vi "Ximea Camera Engine.vi"(0 "Ximea Notifier Name":string, 11 "Camera ID":string[](array[string])) -> ()   [LabVIEW 2016]
uses:
  Ximea Controls/Ximea ROI.ctl
  Ximea Controls/Ximea Parameters.ctl
  Ximea Controls/Ximea Parameter List.ctl
  xiLIB_64bit/xiLIB/xiCamLib/xiCam/PRM/PRM/PRM_v2.ctl
  Ximea Controls/Ximea Notifier Element.ctl
  Ximea Controls/Ximea Actions.ctl
  <vilib>/vision/Image Controls.llb/IMAQ Image.ctl
  Camera Controls/Camera IMAQ Key Info.ctl
panel:
  in  "Use Display Module":bool
  in  "Quit":bool
  in  "Record":bool
  in  "Preview":bool
  out "Acquisition Loop":i32
  in  "Get Param":bool
  in  "Set Param":bool
  in  "Ximea  Parameter":T1
  in  "Get ROI":bool
  in  "Set ROI":bool
  in  "ROI Setup":T3
  out "Acquisition Frame":u32
  out "Serial No.":string
  out "Device Name":string
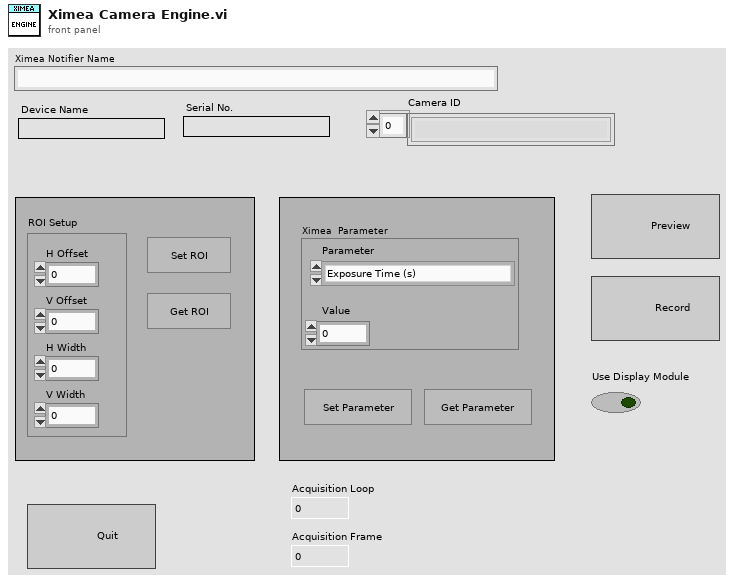
[diagram p1: front panel]
types:
  T1 = typedef "Ximea Parameters.ctl" = cluster{"Parameter":T2, "Value":sgl}
  T2 = typedef "Ximea Parameter List.ctl" = enum16{"Exposure Time (s)", "Gain"}
  T3 = typedef "Ximea ROI.ctl" = cluster{"H Offset":i32, "V Offset":i32, "H Width":i32, "V Width":i32}
  T4 = typedef "PRM_v2.ctl" = enum16{"ACQ_BUFFER_SIZE", "ACQ_FRAME_BURST_COUNT", "ACQ_TIMING_MODE", "ACQ_TRANSPORT_BUFFER_SIZE", "AE_MAX_LIMIT", "AEAG", "AEAG_LEVEL", "API_VERSION", "AG_MAX_LIMIT", "APPLY_CMS", "AUTO_BANDWIDTH_CALCULATION", "AUTO_WB", "AVAILABLE_BANDWIDTH", "AVAILABLE_BANDWIDTH_MAX", "AVAILABLE_BANDWIDTH_MIN", "BUFFER_POLICY", "BUFFERS_QUEUE_SIZE", "CC_MATRIX_00", "CC_MATRIX_01", "CC_MATRIX_02", "CC_MATRIX_03", "CC_MATRIX_10", "CC_MATRIX_11", "CC_MATRIX_12", "CC_MATRIX_13", "CC_MATRIX_20", "CC_MATRIX_21", "CC_MATRIX_22", "CC_MATRIX_23", "CC_MATRIX_30", "CC_MATRIX_31", "CC_MATRIX_32", "CC_MATRIX_33", "CHIP_TEMP", "CMS", "COLOR_FILTER_ARRAY", "COOLING", "DEBOUNCE_EN", "DEBOUNCE_POL", "DEBOUNCE_T0", "DEBOUNCE_T1", "DEBUG_LEVEL", "DEFAULT_CC_MATRIX", "DEVICE_INSTANCE_PATH", "DEVICE_MODEL_ID", "DEVICE_NAME", "DEVICE_SN", "DEVICE_TYPE", "DEVICE_USER_ID", "DOWNSAMPLING", "DOWNSAMPLING_TYPE", "DRV_VERSION", "EXP_PRIORITY", "EXPOSURE", "EXPOSURE_MAX", "EXPOSURE_MIN", "FFS_FILE_NAME", "FPGA1_VERSION", "FRAMERATE", "FRAMERATE_MAX", "FRAMERATE_MIN", "FREE_FFS_SIZE", "GAIN", "GAIN_MAX", "GAIN_MIN", "GAMMAC", "GAMMAY", "GPI_LEVEL", "GPI_MODE", "GPI_SELECTOR", "GPO_MODE", "GPO_SELECTOR", "HDR", "HDR_T1", "HDR_T2", "HEIGHT", "HEIGHT_MAX", "HEIGHT_MIN", "HOUSE_TEMP", "IMAGE_DATA_FORMAT", "IMAGE_IS_COLOR", "INPUT_CMS_PROFILE", "IS_COOLED", "IS_DEVICE_EXIST", "KNEEPOINT1", "KNEEPOINT2", "LED_MODE", "LED_SELECTOR", "LIMIT_BANDWIDTH", "LIMIT_BANDWIDTH_MAX", "LIMIT_BANDWIDTH_MIN", "LUT_EN", "LUT_INDEX", "LUT_INDEX_MAX", "LUT_INDEX_MIN", "LUT_VALUE", "LUT_VALUE_MAX", "LUT_VALUE_MIN", "MANUAL_WB", "MCU1_VERSION", "MCU2_VERSION", "OFFSET_X", "OFFSET_X_MAX", "OFFSET_X_MIN", "OFFSET_Y", "OFFSET_Y_MAX", "OFFSET_Y_MIN", "OUTPUT_CMS_PROFILE", "OUTPUT_DATA_BIT_DEPTH", "OUTPUT_DATA_PACKING", "READ_FILE_FFS", "RECENT_FRAME", "SENSOR_DATA_BIT_DEPTH", "SENSOR_MODE", "SENSOR_TAPS", "SHARPNESS", "SHUTTER_TYPE", "TARGET_TEMP", "TRG_DELAY", "TRG_SELECTOR", "TRG_SOFTWARE", "TRG_SOURCE", "USED_FFS_SIZE", "WB_KB", "WB_KG", "WB_KR", "WIDTH", "WIDTH_MAX", "WIDTH_MIN", "WRITE_FILE_FFS", "ACQ_BUFFER_SIZE_UNIT", "ACQ_TRANSPORT_BUFFER_COMMIT", "AEAG_ROI_HEIGHT", "AEAG_ROI_OFFSET_X", "AEAG_ROU_OFFSET_Y", "AEAG_ROI_WIDTH", "API_CONTEXT_LIST", "BINNING_HORIZONTAL", "BINNING_SELECTOR", "BINNING_VERTICAL", "COLUMN_FPN_CORRECTION", "COUNTER_SELECTOR", "COUNTER_VALUE", "DECIMATION_HORIZONTAL", "DECIMATION_SELECTOR", "DECIMATION_VERTICAL", "DEVICE_ID", "DEVICE_LOCATION_PATH", "DEVICE_MANIFEST", "DEVICE_RESET", "DEVICE_SENS_SN", "EXPOSURE_BURST_COUNT", "FFS_ACCESS_KEY", "GAIN_SELECTOR", "HW_REVISION", "IMAGE_BLACK_LEVEL", "IMAGE_DATA_BIT_DEPTH", "IMAGE_DATA_FORMAT_RGB32_ALPHA", "IMAGE_PAYLOAD_SIZE", "LENS_APERTURE_VALUE", "LENS_FEATURE", "LENS_FEATURE_SELECTOR", "LENS_FOCAL_LENGTH", "LENS_FOCUS_DISTANCE", "LENS_FOCUS_MOVE", "LENS_FOCUS_MOVEMENT_VALUE", "LENS_MODE", "OUTPUT_DATA_PACKING_TYPE", "SENSOR_CLOCK_FREQ_HZ", "SENSOR_CLOCK_FREQ_INDEX", "SENSOR_FEATURE_SELECTOR", "SENSOR_FEATURE_VALUE", "SENSOR_OUTPUT_CHANNEL_COUNT", "TRANSPORT_PIXEL_FORMAT", "TS_RST_MODE", "TS_RST_SOURCE", "SENS_DEFECTS_CORR_LIST_SELECTOR", "SENS_DEFECTS_CORR", "SENS_DEFECTS_CORR_LIST_CONTENT", "DEVICE_UNIT_SELECTOR", "DEVICE_UNIT_REGISTER_SELECTOR", "DEVICE_UNIT_REGISTER_VALUE"}
  T5 = typedef "Camera IMAQ Key Info.ctl" = cluster{"Frame":u32, "Sensor Height":i32, "Sensor Width":i32, "ROI Height":i32, "ROI Width":i32, "ROI Enable?":bool, "Bit per Pixel":u8}
  T6 = typedef "Image Type" = u32
  T7 = typedef "Ximea Notifier Element.ctl" = cluster{"Ximea Actions":T8, "Received?":bool, "Ximea Parameter":T1, "Ximea ROI":T3, "Running?":bool, "File Path":path, "# of frames":u32, "Image Ref":T9, "Error":errorcluster, "Trigger?":bool, "ROI Increment":i32}
  T8 = typedef "Ximea Actions.ctl" = enum16{"Idle", "Error Check", "Preview", "Record", "Soft Trigger", "Abort", "Record Settings", "Set Parameter", "Get Parameter", "Set ROI", "Get ROI", "Status", "Quit"}
  T9 = typedef "IMAQ Image.ctl" = refnum<image>
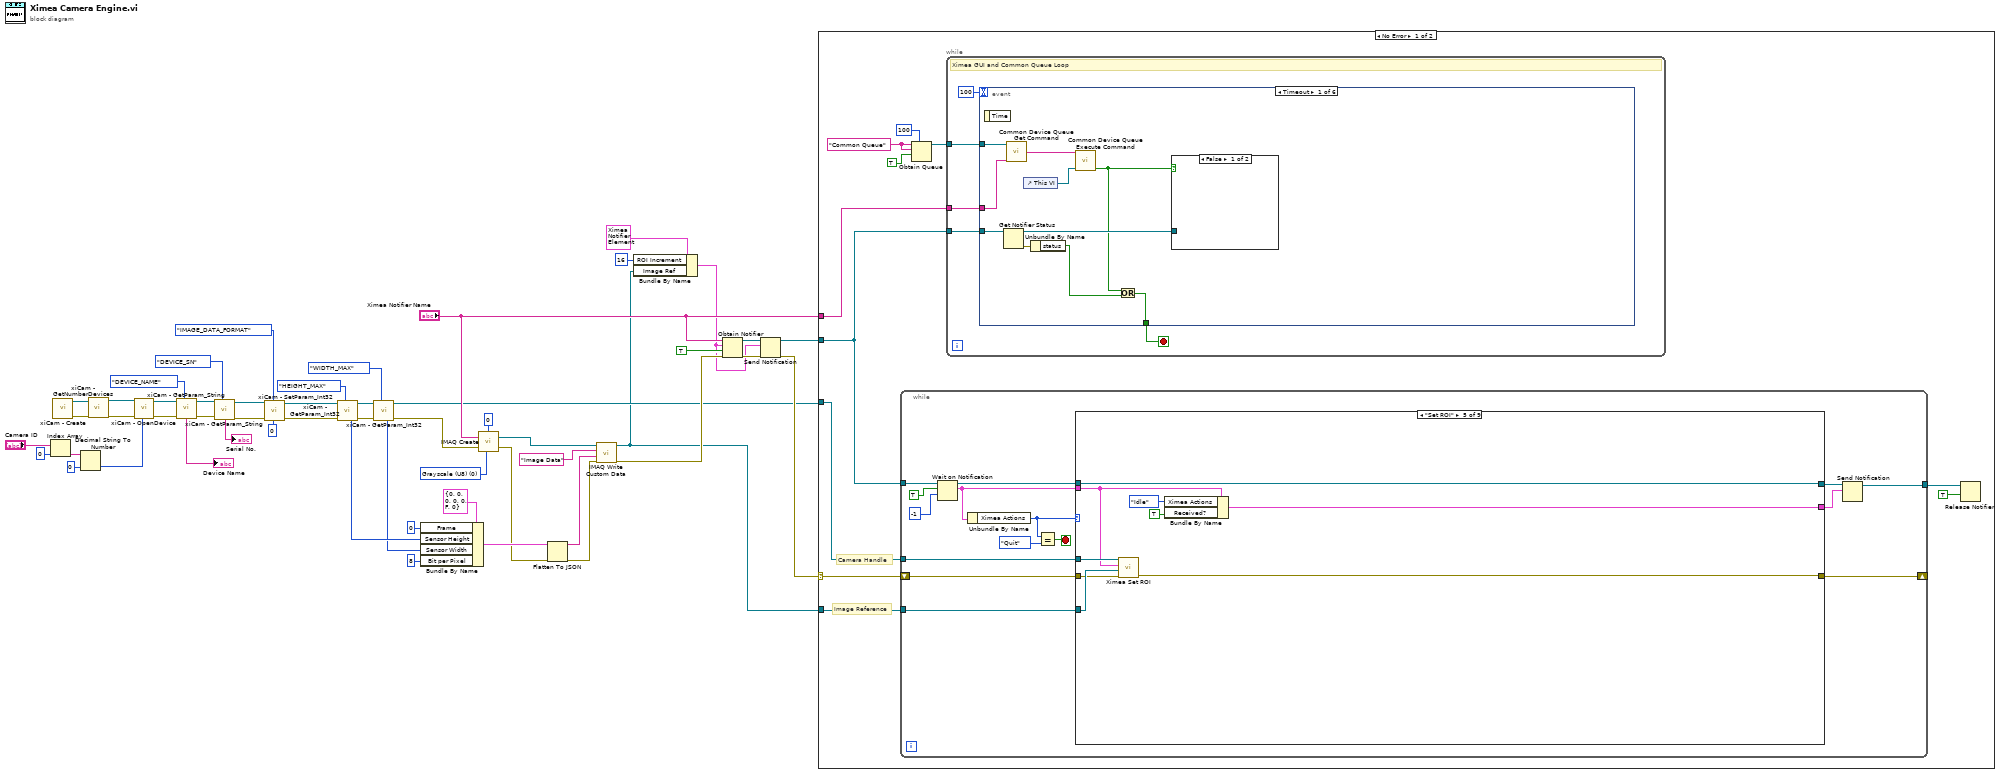
[diagram p0: block diagram]
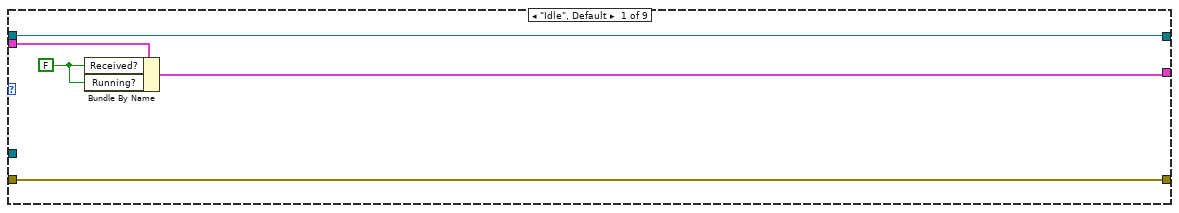
[diagram p2: hidden frame]
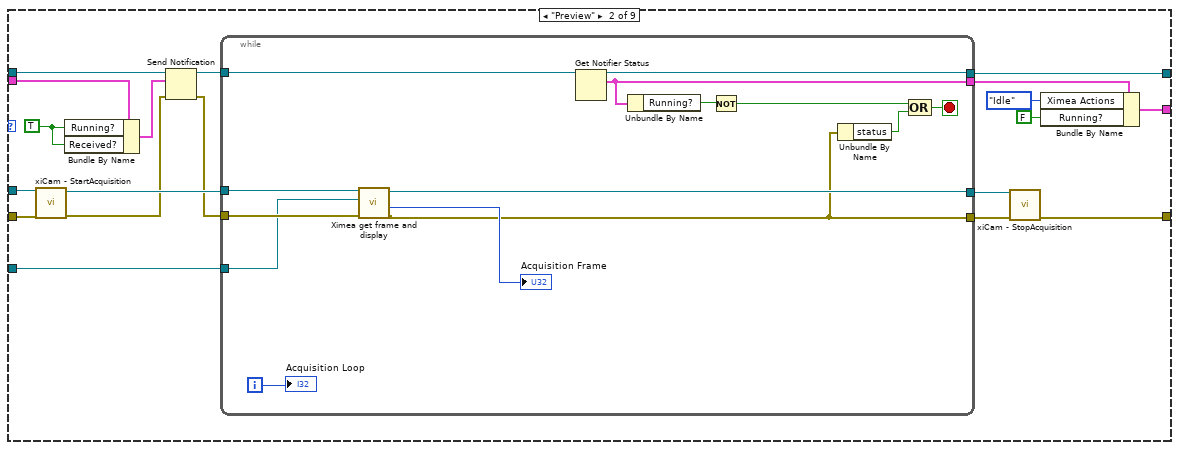
[diagram p3: hidden frame]
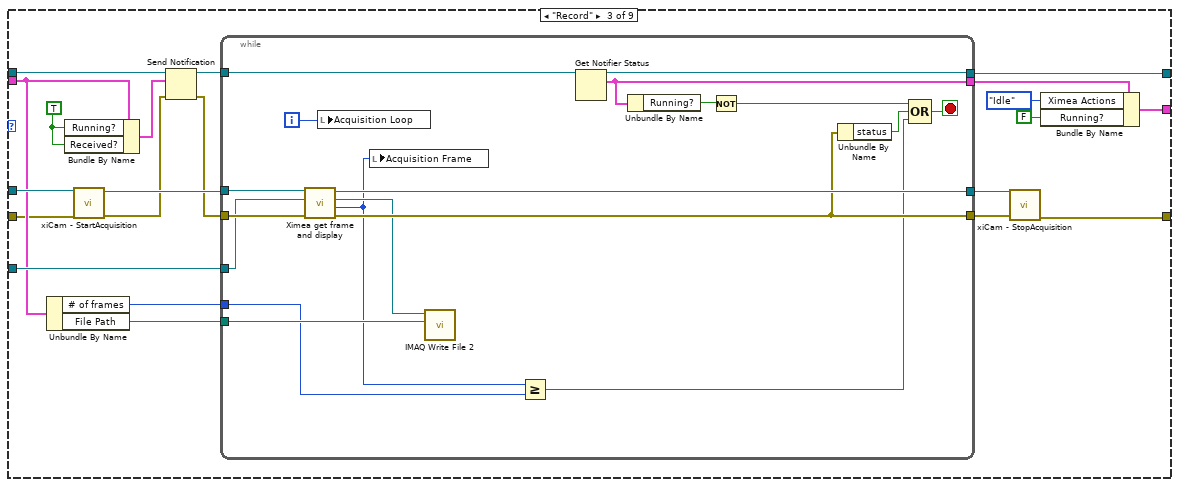
[diagram p4: hidden frame]
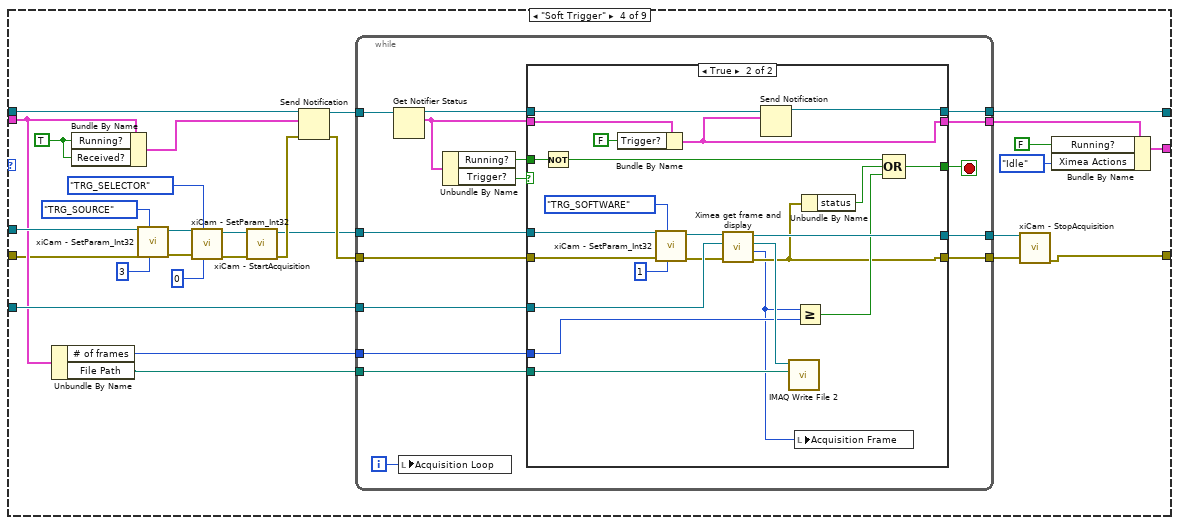
[diagram p5: hidden frame]
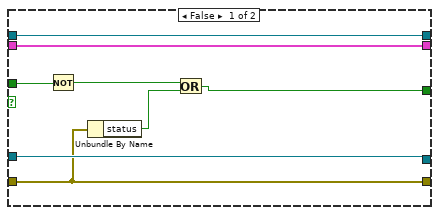
[diagram p6: hidden frame]
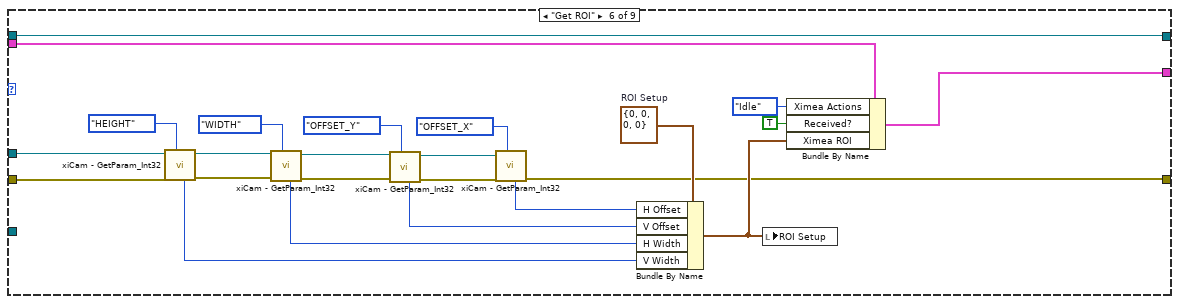
[diagram p7: hidden frame]
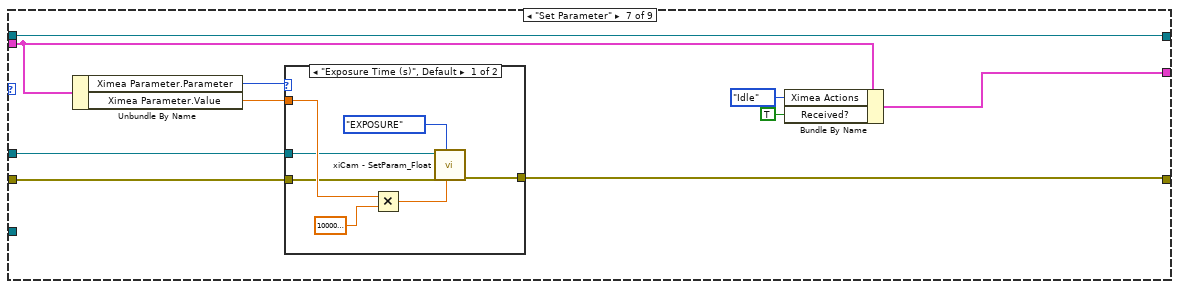
[diagram p8: hidden frame]
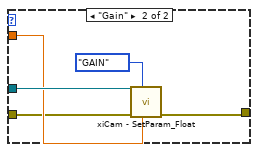
[diagram p9: hidden frame]
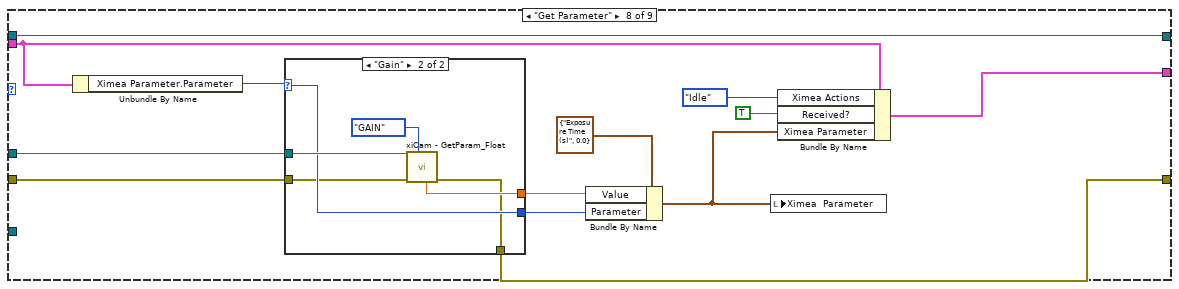
[diagram p10: hidden frame]
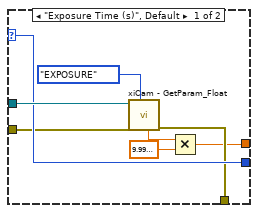
[diagram p11: hidden frame]
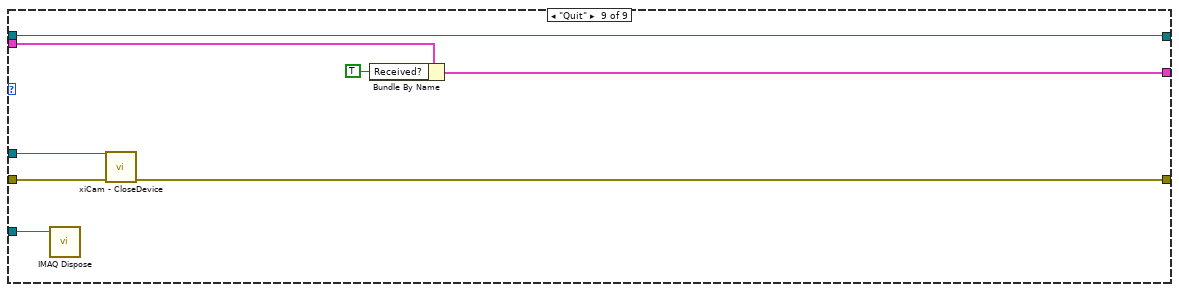
[diagram p12: hidden frame]
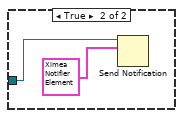
[diagram p13: hidden frame]
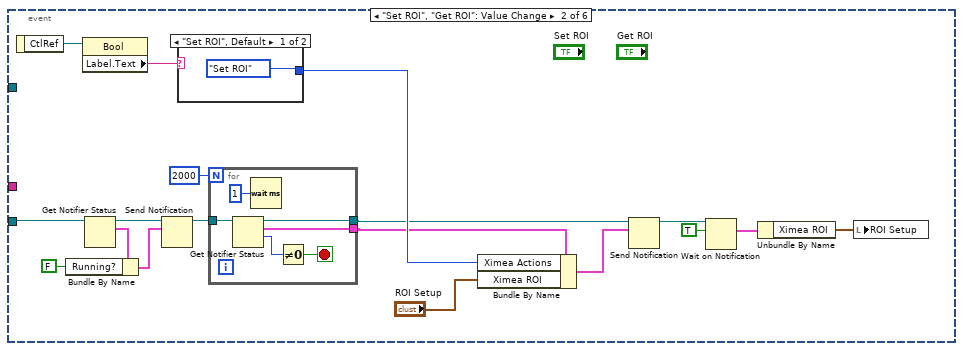
[diagram p14: hidden frame]
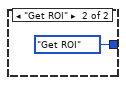
[diagram p15: hidden frame]
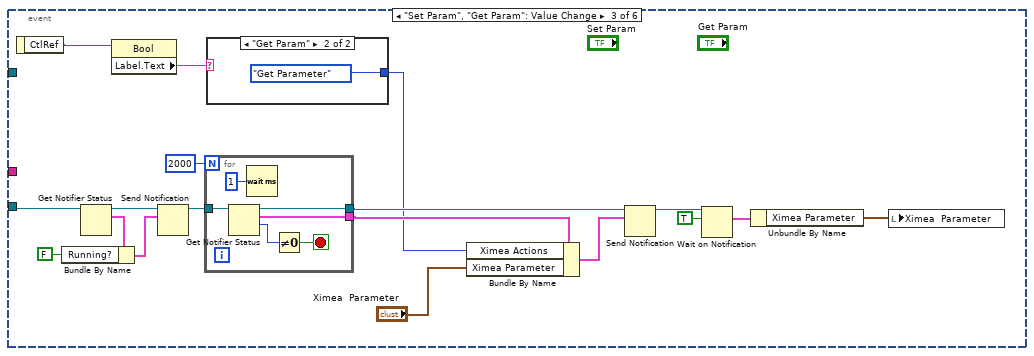
[diagram p16: hidden frame]
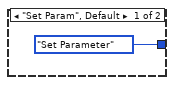
[diagram p17: hidden frame]
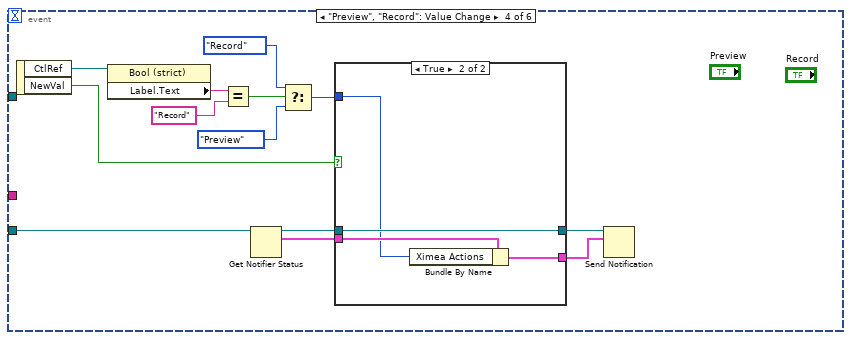
[diagram p18: hidden frame]
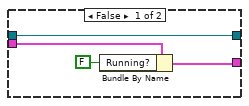
[diagram p19: hidden frame]
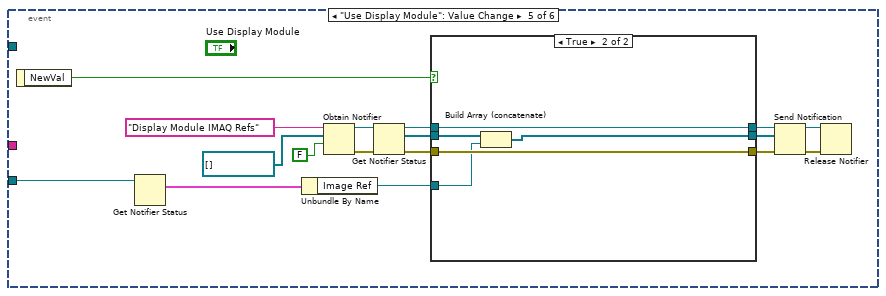
[diagram p20: hidden frame]
diagram:
  w35 = T6 0 items=["Grayscale (U8)", "Grayscale (I16)", "Grayscale (SGL)", "Complex (CSG)", "RGB (U32)", "HSL (U32)", "RGB (U64)", "Grayscale (U16)"] ("Image Type")
  n1 = Index Array(array="Camera ID", index=0) -> (element=w12:string)
  n2 = call "xiCam - Create.vi"() -> ("error out"=w51:errorcluster, "new xiCam"=w53:refnum<k24>)  [unwired: 10 in]
  n3 = Decimal String To Number(string=w12, default (0L)=u32 0 ("default (0 I32)")) -> (number=w10:u32)  [unwired: 1 in, 1 out]
  n4 = call "xiCam - GetNumberDevices.vi"("error in (no error)"=w51, "xiCam In"=w53) -> ("error out"=w50:errorcluster, "xiCam Out"=w52:refnum<k24>)  [unwired: 7 in, 1 out]
  n5 = call "xiCam - OpenDevice.vi"("DevID"=w10, "error in (no error)"=w50, "xiCam In"=w52) -> ("error out"=w22:errorcluster, "xiCam Out"=w30:refnum<k24>)  [unwired: 7 in]
  n6 = call "xiCam - GetParam_String.vi"("PRM"=PRM_v2."DEVICE_NAME", "error in (no error)"=w22, "xiCam In"=w30) -> ("error out"=w21:errorcluster, "xiCam Out"=w47:refnum<k24>, "String_Value"=→"Device Name":string)  [unwired: 6 in]
  n7 = call "xiCam - GetParam_String.vi"("PRM"=PRM_v2."DEVICE_SN", "error in (no error)"=w21, "xiCam In"=w47) -> ("error out"=w15:errorcluster, "xiCam Out"=w16:refnum<k24>, "String_Value"=→"Serial No.":string)  [unwired: 6 in]
  n8 = call "xiCam - SetParam_Int32.vi"("Int32_Value"=0, "PRM"=PRM_v2."IMAGE_DATA_FORMAT", "error in (no error)"=w15, "xiCam In"=w16) -> ("error out"=w9:errorcluster, "xiCam Out"=w8:refnum<k24>)  [unwired: 6 in]
  n9 = call "xiCam - GetParam_Int32.vi"("PRM"=PRM_v2."HEIGHT_MAX", "error in (no error)"=w9, "xiCam In"=w8) -> ("error out"=w6:errorcluster, "xiCam Out"=w7:refnum<k24>, "Int32_Value"=w31:i32)  [unwired: 6 in]
  n10 = call "xiCam - GetParam_Int32.vi"("PRM"=PRM_v2."WIDTH_MAX", "error in (no error)"=w6, "xiCam In"=w7) -> ("error out"=w5:errorcluster, "xiCam Out"=w4:refnum<k24>, "Int32_Value"=w28:i32)  [unwired: 6 in]
  n11 = Bundle By Name(cluster=T5 {"Frame"=0, "Sensor Height"=0, "Sensor Width"=0, "ROI Height"=0, "ROI Width"=0, "ROI Enable?"=FALSE, "Bit per Pixel"=0} ("Camera IMAQ Key Info"), "Frame"=u32 0, "Sensor Height"=w31, "Sensor Width"=w28, "Bit per Pixel"=u8 8) -> (w41:T5)
  n12 = call "IMAQ Create"("Border Size"=0, "Image Name"="Ximea Notifier Name", "Image Type"=w35, "error in (no error)"=w5) -> ("New Image"=w37:T9, "error out"=w34:errorcluster)  [unwired: 1 in]
  n13 = Flatten To JSON(anything=w41, error in (no error)=w34) -> (JSON string=w42:string, 11:w33:errorcluster)  [unwired: 1 in]
  n14 = call "IMAQ Write Custom Data"("error in (no error)"=w33, "Custom Data In"=w42, "Key"="Image Data", "Image"=w37) -> ("error out"=w26:errorcluster, "Image Out"=w2:T9)  [unwired: 6 in]
  n15 = Bundle By Name(cluster=T7 {"Ximea Actions"=enum."Error Check", "Received?"=FALSE, "Ximea Parameter"={"Parameter"=enum."Exposure Time (s)", "Value"=0.0}, "Ximea ROI"={"H Offset"=0, "V Offset"=0, "H Width"=0, "V Width"=0}, "Running?"=FALSE, "File Path"=path "", "# of frames"=0, "Image Ref"=refnum, "Error"={"status"=FALSE, "code"=0, "source"=""}, "Trigger?"=FALSE, "ROI Increment"=0} ("Ximea Camera Cluster"), "ROI Increment"=16, "Image Ref"=w2) -> (w3:T7)
  n16 = Obtain Notifier(name (unnamed)="Ximea Notifier Name", notification data type=w3, create if not found? (T)=TRUE, error in (no error)=w26) -> (notifier out=w44:refnum<notifier>, error out=w25:errorcluster)  [unwired: 1 out]
  n17 = Send Notification(notification=w3, notifier=w44, error in (no error)=w25) -> (notifier out=w24:refnum<notifier>, error out=w20:errorcluster)
  n18 = case shown="No Error" w20 {
    selector: w20 -> [w56 w461]
    tunnel: "Ximea Notifier Name" -> [w64 w463]
    tunnel: w24 -> [w59 w462]
    tunnel: w4 -> [w58 w459]
    tunnel: w2 -> [w57 w456]
    frame No Error {
      w63 = "Common Queue" ("Unique Notifier Name")
      # "Image Reference"
      # "Camera Handle"
      n19 = while {
        tunnel: w59 -> [w79]
        tunnel: w58 -> [w71]
        tunnel: w57 -> [w65]
        tunnel: [w68] -> w54
        shift-right: [w66] -> _
        shift-left: w56 -> [w67]
        stop <- w72 stop-if-true
        n20 = Wait on Notification(notifier=w79, ignore previous (F)=TRUE, timeout in ms (-1)=-1) -> (notifier out=w76:refnum<notifier>, notification=w75:T7)  [unwired: 1 in, 2 out]
        n21 = Unbundle By Name(w75) -> ("Ximea Actions"=w74:T8)
        n22 = Equal?(x=w74, y=Ximea_Actions."Quit") -> (x = y?=w72:bool)
        n23 = case shown="\"Set ROI\"" w74 {
          tunnel: w76 -> [w82 w100 w135 w177 w241 w253 w272 w298 w319]
          tunnel: w75 -> [w84 w98 w122 w168 w236 w251 w271 w297 w318]
          tunnel: w71 -> [_ w102 w137 w183 w237 w261 w273 w299 w322]
          tunnel: w65 -> [_ w103 w138 w169 w235 _ _ _ w315]
          tunnel: [w82 w89 w125 w163 w241 w253 w272 w298 w319] -> w70
          tunnel: [w81 w88 w124 w161 w238 w247 w268 w294 w316] -> w69
          tunnel: w67 -> [w80 w85 w118 w157 w234 w246 w267 w289 w321]
          tunnel: [w80 w86 w119 w158 w233 w242 w266 w288 w320] -> w66
          frame "Idle", Default {
            w83 = FALSE ("Received?")
            n24 = Bundle By Name(cluster=w84, "Received?"=w83, "Running?"=w83) -> (w81:T7)
          }
          frame "Preview" {
            w97 = TRUE ("Received?")
            n25 = call "xiCam - StartAcquisition.vi"("error in (no error)"=w85, "xiCam In"=w102) -> ("error out"=w95:errorcluster, "xiCam Out"=w101:refnum<k24>)  [unwired: 8 in]
            n26 = Bundle By Name(cluster=w98, "Running?"=w97, "Received?"=w97) -> (w96:T7)
            n27 = Send Notification(notification=w96, notifier=w100, error in (no error)=w95) -> (notifier out=w99:refnum<notifier>, error out=w94:errorcluster)
            n28 = while {
              tunnel: w101 -> [w110]
              tunnel: w103 -> [w108]
              tunnel: w99 -> [w117]
              tunnel: w94 -> [w109]
              tunnel: [w116] -> w89
              tunnel: [w112] -> w91
              tunnel: [w106] -> w93
              tunnel: [w105] -> w92
              i -> [w104]
              stop <- w111 stop-if-true
              n29 = call "Ximea get frame and display.vi"("error in (no error)"=w109, "Image In"=w108, "xiCam In"=w110) -> ("error out"=w105:errorcluster, "FrameNumber"=→"Acquisition Frame":u32, "xiCam Out"=w106:refnum<k24>)  [unwired: 5 in, 1 out]
              n30 = Get Notifier Status(notifier=w117) -> (notifier out=w116:refnum<notifier>, current notification=w112:T7)  [unwired: 1 in, 3 out]
              n31 = Unbundle By Name(w112) -> ("Running?"=w115:bool)
              n32 = Not(x=w115) -> (.not. x?=w114:bool)
              n33 = Unbundle By Name(w105) -> ("status"=w113:bool)
              n34 = Compound Arithmetic op=OR(w114, w113) -> (w111:bool)
              "Acquisition Loop" <- w104
            }
            n35 = call "xiCam - StopAcquisition.vi"("error in (no error)"=w92, "xiCam In"=w93) -> ("error out"=w86:errorcluster)  [unwired: 8 in, 1 out]
            n36 = Bundle By Name(cluster=w91, "Ximea Actions"=Ximea_Actions."Idle", "Running?"=FALSE) -> (w88:T7)
          }
          frame "Record" {
            w133 = TRUE ("Received?")
            n37 = Unbundle By Name(w122) -> ("# of frames"=w121:u32, "File Path"=w120:path)
            n38 = Bundle By Name(cluster=w122, "Running?"=w133, "Received?"=w133) -> (w132:T7)
            n39 = call "xiCam - StartAcquisition.vi"("error in (no error)"=w118, "xiCam In"=w137) -> ("error out"=w131:errorcluster, "xiCam Out"=w136:refnum<k24>)  [unwired: 8 in]
            n40 = Send Notification(notification=w132, notifier=w135, error in (no error)=w131) -> (notifier out=w134:refnum<notifier>, error out=w130:errorcluster)
            n41 = while {
              tunnel: w136 -> [w156]
              tunnel: w138 -> [w154]
              tunnel: w134 -> [w153]
              tunnel: w130 -> [w155]
              tunnel: [w152] -> w125
              tunnel: [w148] -> w127
              tunnel: [w146] -> w129
              tunnel: [w145] -> w128
              tunnel: w121 -> [w142]
              tunnel: w120 -> [w143]
              i -> [w144]
              stop <- w147 stop-if-true
              n42 = call "Ximea get frame and display.vi"("error in (no error)"=w155, "Image In"=w154, "xiCam In"=w156) -> ("error out"=w145:errorcluster, "FrameNumber"=w139:u32, "Image Out"=w140:T9, "xiCam Out"=w146:refnum<k24>)  [unwired: 5 in]
              n43 = local write "Acquisition Loop"(w144) -> ()
              n44 = local write "Acquisition Frame"(w139) -> ()
              n45 = call-poly "IMAQ Write File 2"("File Path"=w143, "Image"=w140) -> ()  [unwired: 8 in, 2 out]
              n46 = Greater Or Equal?(x=w139, y=w142) -> (x >= y?=w141:bool)
              n47 = Get Notifier Status(notifier=w153) -> (notifier out=w152:refnum<notifier>, current notification=w148:T7)  [unwired: 1 in, 3 out]
              n48 = Unbundle By Name(w148) -> ("Running?"=w151:bool)
              n49 = Not(x=w151) -> (.not. x?=w150:bool)
              n50 = Unbundle By Name(w145) -> ("status"=w149:bool)
              n51 = Compound Arithmetic op=OR(w150, w149, w141) -> (w147:bool)
            }
            n52 = call "xiCam - StopAcquisition.vi"("error in (no error)"=w128, "xiCam In"=w129) -> ("error out"=w119:errorcluster)  [unwired: 8 in, 1 out]
            n53 = Bundle By Name(cluster=w127, "Ximea Actions"=Ximea_Actions."Idle", "Running?"=FALSE) -> (w124:T7)
          }
          frame "Soft Trigger" {
            w178 = TRUE ("Running?")
            n54 = Unbundle By Name(w168) -> ("# of frames"=w166:u32, "File Path"=w167:path)
            n55 = Bundle By Name(cluster=w168, "Running?"=w178, "Received?"=w178) -> (w176:T7)
            n56 = call "xiCam - SetParam_Int32.vi"("Int32_Value"=3, "PRM"=PRM_v2."TRG_SOURCE", "error in (no error)"=w157, "xiCam In"=w183) -> ("error out"=w175:errorcluster, "xiCam Out"=w182:refnum<k24>)  [unwired: 6 in]
            n57 = call "xiCam - SetParam_Int32.vi"("Int32_Value"=0, "PRM"=PRM_v2."TRG_SELECTOR", "error in (no error)"=w175, "xiCam In"=w182) -> ("error out"=w174:errorcluster, "xiCam Out"=w179:refnum<k24>)  [unwired: 6 in]
            n58 = call "xiCam - StartAcquisition.vi"("error in (no error)"=w174, "xiCam In"=w179) -> ("error out"=w173:errorcluster, "xiCam Out"=w170:refnum<k24>)  [unwired: 8 in]
            n59 = Send Notification(notification=w176, notifier=w177, error in (no error)=w173) -> (notifier out=w171:refnum<notifier>, error out=w172:errorcluster)
            n60 = while {
              tunnel: w172 -> [w197]
              tunnel: w171 -> [w201]
              tunnel: w170 -> [w199]
              tunnel: w169 -> [w198]
              tunnel: [w196] -> w165
              tunnel: w167 -> [w195]
              tunnel: w166 -> [w194]
              tunnel: [w190] -> w163
              tunnel: [w189] -> w162
              tunnel: [w188] -> w164
              i -> [w186]
              stop <- w187 stop-if-true
              n61 = Get Notifier Status(notifier=w201) -> (notifier out=w193:refnum<notifier>, current notification=w192:T7)  [unwired: 1 in, 3 out]
              n62 = local write "Acquisition Loop"(w186) -> ()
              n63 = Unbundle By Name(w192) -> ("Running?"=w191:bool, "Trigger?"=w200:bool)
              n64 = case shown="True" w200 {
                tunnel: w199 -> [w207 w232]
                tunnel: w198 -> [_ w228]
                tunnel: w197 -> [w204 w226]
                tunnel: [w207 w225] -> w196
                tunnel: w195 -> [_ w223]
                tunnel: w194 -> [_ w222]
                tunnel: w193 -> [w209 w218]
                tunnel: w192 -> [w208 w221]
                tunnel: w191 -> [w206 w219]
                tunnel: [w209 w217] -> w190
                tunnel: [w208 w212] -> w189
                tunnel: [w204 w211] -> w188
                tunnel: [w202 w213] -> w187
                frame False {
                  n65 = Not(x=w206) -> (.not. x?=w205:bool)
                  n66 = Unbundle By Name(w204) -> ("status"=w203:bool)
                  n67 = Or(x=w205, y=w203) -> (x .or. y?=w202:bool)
                }
                frame True {
                  n68 = Not(x=w219) -> (.not. x?=w216:bool)
                  n69 = Bundle By Name(cluster=w221, "Trigger?"=FALSE) -> (w212:T7)
                  n70 = call "xiCam - SetParam_Int32.vi"("Int32_Value"=1, "PRM"=PRM_v2."TRG_SOFTWARE", "error in (no error)"=w226, "xiCam In"=w232) -> ("error out"=w227:errorcluster, "xiCam Out"=w229:refnum<k24>)  [unwired: 6 in]
                  n71 = call "Ximea get frame and display.vi"("error in (no error)"=w227, "Image In"=w228, "xiCam In"=w229) -> ("error out"=w211:errorcluster, "FrameNumber"=w210:u32, "Image Out"=w224:T9, "xiCam Out"=w225:refnum<k24>)  [unwired: 5 in]
                  n72 = Send Notification(notification=w212, notifier=w218) -> (notifier out=w217:refnum<notifier>)  [unwired: 1 in, 1 out]
                  n73 = call-poly "IMAQ Write File 2"("File Path"=w223, "Image"=w224) -> ()  [unwired: 8 in, 2 out]
                  n74 = Greater Or Equal?(x=w210, y=w222) -> (x >= y?=w214:bool)
                  n75 = local write "Acquisition Frame"(w210) -> ()
                  n76 = Unbundle By Name(w211) -> ("status"=w215:bool)
                  n77 = Compound Arithmetic op=OR(w216, w215, w214) -> (w213:bool)
                }
              }
            }
            n78 = call "xiCam - StopAcquisition.vi"("error in (no error)"=w164, "xiCam In"=w165) -> ("error out"=w158:errorcluster)  [unwired: 8 in, 1 out]
            n79 = Bundle By Name(cluster=w162, "Running?"=FALSE, "Ximea Actions"=Ximea_Actions."Idle") -> (w161:T7)
          }
          frame "Set ROI" {
            n80 = call "Ximea Set ROI.vi"("error in"=w234, "Image Ref"=w235, "Ximea Camera Cluster"=w236, "xiCam In"=w237) -> ("error out"=w233:errorcluster)  [unwired: 6 in, 1 out]
            n81 = Bundle By Name(cluster=w236, "Ximea Actions"=Ximea_Actions."Idle", "Received?"=TRUE) -> (w238:T7)
          }
          frame "Get ROI" {
            w252 = T3 {"H Offset"=0, "V Offset"=0, "H Width"=0, "V Width"=0}  # ROI Setup
            n82 = call "xiCam - GetParam_Int32.vi"("PRM"=PRM_v2."HEIGHT", "error in (no error)"=w246, "xiCam In"=w261) -> ("error out"=w245:errorcluster, "xiCam Out"=w256:refnum<k24>, "Int32_Value"=w257:i32)  [unwired: 6 in]
            n83 = call "xiCam - GetParam_Int32.vi"("PRM"=PRM_v2."WIDTH", "error in (no error)"=w245, "xiCam In"=w256) -> ("error out"=w244:errorcluster, "xiCam Out"=w255:refnum<k24>, "Int32_Value"=w258:i32)  [unwired: 6 in]
            n84 = call "xiCam - GetParam_Int32.vi"("PRM"=PRM_v2."OFFSET_Y", "error in (no error)"=w244, "xiCam In"=w255) -> ("error out"=w243:errorcluster, "xiCam Out"=w254:refnum<k24>, "Int32_Value"=w259:i32)  [unwired: 6 in]
            n85 = call "xiCam - GetParam_Int32.vi"("PRM"=PRM_v2."OFFSET_X", "error in (no error)"=w243, "xiCam In"=w254) -> ("error out"=w242:errorcluster, "Int32_Value"=w260:i32)  [unwired: 6 in, 1 out]
            n86 = Bundle By Name(cluster=w252, "H Offset"=w260, "V Offset"=w259, "H Width"=w258, "V Width"=w257) -> (w250:T3)
            n87 = local write "ROI Setup"(w250) -> ()
            n88 = Bundle By Name(cluster=w251, "Ximea Actions"=Ximea_Actions."Idle", "Received?"=TRUE, "Ximea ROI"=w250) -> (w247:T7)
          }
          frame "Set Parameter" {
            n89 = Unbundle By Name(w271) -> ("Ximea Parameter.Parameter"=w275:T2, "Ximea Parameter.Value"=w274:sgl)
            n90 = case shown="\"Exposure Time (s)\", Default" w275 {
              tunnel: w274 -> [w281 w285]
              tunnel: w273 -> [w280 w287]
              tunnel: w267 -> [w277 w284]
              tunnel: [w276 w283] -> w266
              frame "Exposure Time (s)", Default {
                n91 = Multiply(x=w281, y=sgl 1000000.0) -> (x*y=w278:sgl)
                n92 = call "xiCam - SetParam_Float.vi"("Float_Value"=w278, "PRM"=PRM_v2."EXPOSURE", "error in (no error)"=w277, "xiCam In"=w280) -> ("error out"=w276:errorcluster)  [unwired: 6 in, 1 out]
              }
              frame "Gain" {
                n93 = call "xiCam - SetParam_Float.vi"("Float_Value"=w285, "PRM"=PRM_v2."GAIN", "error in (no error)"=w284, "xiCam In"=w287) -> ("error out"=w283:errorcluster)  [unwired: 6 in, 1 out]
              }
            }
            n94 = Bundle By Name(cluster=w271, "Ximea Actions"=Ximea_Actions."Idle", "Received?"=TRUE) -> (w268:T7)
          }
          frame "Get Parameter" {
            n95 = Unbundle By Name(w297) -> ("Ximea Parameter.Parameter"=w300:T2)
            n96 = case shown="\"Gain\"" w300 {
              selector: w300 -> [w306 w311]
              tunnel: w299 -> [w308 w314]
              tunnel: [w301 w312] -> w292
              tunnel: [w306 w311] -> w291
              tunnel: w289 -> [w305 w310]
              tunnel: [w304 w309] -> w288
              frame "Exposure Time (s)", Default {
                n97 = call "xiCam - GetParam_Float.vi"("PRM"=PRM_v2."EXPOSURE", "error in (no error)"=w305, "xiCam In"=w308) -> ("error out"=w304:errorcluster, "Float_Value"=w303:sgl)  [unwired: 6 in, 1 out]
                n98 = Multiply(x=w303, y=sgl 1e-06) -> (x*y=w301:sgl)
              }
              frame "Gain" {
                n99 = call "xiCam - GetParam_Float.vi"("PRM"=PRM_v2."GAIN", "error in (no error)"=w310, "xiCam In"=w314) -> ("error out"=w309:errorcluster, "Float_Value"=w312:sgl)  [unwired: 6 in, 1 out]
              }
            }
            n100 = Bundle By Name(cluster=T1 {"Parameter"=enum."Exposure Time (s)", "Value"=0.0} ("Ximea  Parameter"), "Value"=w292, "Parameter"=w291) -> (w290:T1)
            n101 = local write "Ximea  Parameter"(w290) -> ()
            n102 = Bundle By Name(cluster=w297, "Ximea Actions"=Ximea_Actions."Idle", "Received?"=TRUE, "Ximea Parameter"=w290) -> (w294:T7)
          }
          frame "Quit" {
            n103 = call "IMAQ Dispose"("Image"=w315) -> ()  [unwired: 5 in, 1 out]
            n104 = call "xiCam - CloseDevice.vi"("error in (no error)"=w321, "xiCam In"=w322) -> ("error out"=w320:errorcluster)  [unwired: 9 in]
            n105 = Bundle By Name(cluster=w318, "Received?"=TRUE) -> (w316:T7)
          }
        }
        n106 = Send Notification(notification=w69, notifier=w70) -> (notifier out=w68:refnum<notifier>)  [unwired: 1 in, 1 out]
      }
      n107 = Obtain Queue(max queue size (-1, unlimited)=100, name (unnamed)=w63, element data type=w63, create if not found? (T)=TRUE) -> (queue out=w60:refnum<queue>)  [unwired: 1 in, 2 out]
      n108 = while {
        tunnel: w64 -> [w326]
        tunnel: w60 -> [w325]
        tunnel: w59 -> [w324]
        stop <- w323 stop-if-true
        # "Ximea GUI and Common Queue Loop"
        n109 = event shown="[0] Timeout" {
          selector: _ -> [_ _ _ _ _ _]
          dyn-events: _ -> [_ _ _ _ _ _]
          timeout: 100 ("Numeric") -> [_ _ _ _ _ _]
          tunnel: w326 -> [w334 _ _ _ _ _]
          tunnel: w325 -> [w335 _ _ _ _ _]
          tunnel: w324 -> [w333 w346 w370 w396 w414 w453]
          tunnel: [w328 _ _ _ _ w455] -> w323
          event Timeout {
            n110 = event-data() -> ()  [unwired: 1 in, 1 out]
            n111 = Get Notifier Status(notifier=w333) -> (notifier out=w332:refnum<notifier>, error out=w331:errorcluster)  [unwired: 1 in, 3 out]
            n112 = call "Common Device Queue Get Command.vi"("Common Queue"=w335, "Notifier Name"=w334) -> ("Command"=w337:string)  [unwired: 12 in, 1 out]
            n113 = control-ref of="This VI"() -> (w336:refnum<vi>)
            n114 = Unbundle By Name(w331) -> ("status"=w329:bool)
            n115 = call "Common Device Queue Execute Command.vi"("Common Command"=w337, "VI Refnum"=w336) -> ("Quit?"=w330:bool)  [unwired: 12 in, 1 out]
            n116 = Or(x=w330, y=w329) -> (x .or. y?=w328:bool)
            n117 = case shown="False" w330 {
              tunnel: w332 -> [_ w339]
              frame False {
              }
              frame True {
                n118 = Send Notification(notification=T7 {"Ximea Actions"=enum."Error Check", "Received?"=FALSE, "Ximea Parameter"={"Parameter"=enum."Exposure Time (s)", "Value"=0.0}, "Ximea ROI"={"H Offset"=0, "V Offset"=0, "H Width"=0, "V Width"=0}, "Running?"=FALSE, "File Path"=path "", "# of frames"=0, "Image Ref"=refnum, "Error"={"status"=FALSE, "code"=0, "source"=""}, "Trigger?"=FALSE, "ROI Increment"=0} ("Ximea Camera Cluster"), notifier=w339) -> ()  [unwired: 1 in, 2 out]
              }
            }
          }
          event "Set ROI", "Get ROI": Value Change {
            n119 = event-data() -> ("CtlRef"=w357:refnum<vi>)  [unwired: 1 in]
            n120 = property class="Bool"(reference=w357) -> ("Label.Text"=w356:string)  [unwired: 1 in, 2 out]
            n121 = Get Notifier Status(notifier=w346) -> (notifier out=w349:refnum<notifier>, current notification=w352:T7)  [unwired: 1 in, 3 out]
            n122 = Bundle By Name(cluster=w352, "Running?"=FALSE) -> (w348:T7)
            n123 = Send Notification(notification=w348, notifier=w349) -> (notifier out=w347:refnum<notifier>)  [unwired: 1 in, 1 out]
            n124 = case shown="\"Set ROI\", Default" w356 {
              tunnel: [Ximea_Actions."Set ROI" ("Ximea Actions") Ximea_Actions."Get ROI" ("Ximea Actions")] -> w355
              frame "Set ROI", Default {
              }
              frame "Get ROI" {
              }
            }
            n125 = for {
              N: 2000 -> [_]
              tunnel: w347 -> [w362]
              tunnel: [w361] -> w345
              tunnel: [w360] -> w344
              stop <- w358 stop-if-true
              n126 = Get Notifier Status(notifier=w362) -> (notifier out=w361:refnum<notifier>, current notification=w360:T7, # waiting=w359:i32)  [unwired: 1 in, 2 out]
              n127 = Wait (ms)(milliseconds to wait=u32 1) -> ()  [unwired: 1 out]
              n128 = Not Equal To 0?(x=w359) -> (x != 0?=w358:bool)
            }
            n129 = Bundle By Name(cluster=w344, "Ximea Actions"=w355, "Ximea ROI"="ROI Setup") -> (w353:T7)
            n130 = Send Notification(notification=w353, notifier=w345) -> (notifier out=w343:refnum<notifier>)  [unwired: 1 in, 1 out]
            n131 = Wait on Notification(notifier=w343, ignore previous (F)=TRUE) -> (notification=w341:T7)  [unwired: 2 in, 3 out]
            n132 = Unbundle By Name(w341) -> ("Ximea ROI"=w340:T3)
            n133 = local write "ROI Setup"(w340) -> ()
          }
          event "Set Param", "Get Param": Value Change {
            n134 = event-data() -> ("CtlRef"=w382:refnum<vi>)  [unwired: 1 in]
            n135 = Get Notifier Status(notifier=w370) -> (notifier out=w377:refnum<notifier>, current notification=w380:T7)  [unwired: 1 in, 3 out]
            n136 = Bundle By Name(cluster=w380, "Running?"=FALSE) -> (w376:T7)
            n137 = property class="Bool"(reference=w382) -> ("Label.Text"=w383:string)  [unwired: 1 in, 2 out]
            n138 = Send Notification(notification=w376, notifier=w377) -> (notifier out=w375:refnum<notifier>)  [unwired: 1 in, 1 out]
            n139 = for {
              N: 2000 -> [_]
              tunnel: w375 -> [w388]
              tunnel: [w387] -> w374
              tunnel: [w386] -> w373
              stop <- w384 stop-if-true
              n140 = Get Notifier Status(notifier=w388) -> (notifier out=w387:refnum<notifier>, current notification=w386:T7, # waiting=w385:i32)  [unwired: 1 in, 2 out]
              n141 = Wait (ms)(milliseconds to wait=u32 1) -> ()  [unwired: 1 out]
              n142 = Not Equal To 0?(x=w385) -> (x != 0?=w384:bool)
            }
            n143 = case shown="\"Get Param\"" w383 {
              tunnel: [Ximea_Actions."Set Parameter" ("Ximea Actions") Ximea_Actions."Get Parameter" ("Ximea Actions")] -> w369
              frame "Set Param", Default {
              }
              frame "Get Param" {
              }
            }
            n144 = Bundle By Name(cluster=w373, "Ximea Actions"=w369, "Ximea Parameter"="Ximea  Parameter") -> (w381:T7)
            n145 = Send Notification(notification=w381, notifier=w374) -> (notifier out=w372:refnum<notifier>)  [unwired: 1 in, 1 out]
            n146 = Wait on Notification(notifier=w372, ignore previous (F)=TRUE) -> (notification=w367:T7)  [unwired: 2 in, 3 out]
            n147 = Unbundle By Name(w367) -> ("Ximea Parameter"=w366:T1)
            n148 = local write "Ximea  Parameter"(w366) -> ()
          }
          event "Preview", "Record": Value Change {
            n149 = event-data() -> ("CtlRef"=w404:refnum<vi>, "NewVal"=w398:bool)  [unwired: 1 in]
            n150 = property class="Bool (strict)"(reference=w404) -> ("Label.Text"=w403:string)  [unwired: 1 in, 2 out]
            n151 = Equal?(x=w403, y="Record") -> (x = y?=w401:bool)
            n152 = Get Notifier Status(notifier=w396) -> (notifier out=w395:refnum<notifier>, current notification=w394:T7)  [unwired: 1 in, 3 out]
            n153 = Select(t=Ximea_Actions."Record" ("Ximea Actions"), s=w401, f=Ximea_Actions."Preview") -> (s? t:f=w397:T8)
            n154 = case shown="True" w398 {
              tunnel: w397 -> [_ w410]
              tunnel: w395 -> [w408 w412]
              tunnel: w394 -> [w407 w411]
              tunnel: [w408 w412] -> w393
              tunnel: [w405 w409] -> w392
              frame False {
                n155 = Bundle By Name(cluster=w407, "Running?"=FALSE) -> (w405:T7)
              }
              frame True {
                n156 = Bundle By Name(cluster=w411, "Ximea Actions"=w410) -> (w409:T7)
              }
            }
            n157 = Send Notification(notification=w392, notifier=w393) -> ()  [unwired: 1 in, 2 out]
          }
          event "Use Display Module": Value Change {
            n158 = event-data() -> ("NewVal"=w413:bool)  [unwired: 1 in]
            n159 = Get Notifier Status(notifier=w414) -> (current notification=w429:T7)  [unwired: 1 in, 4 out]
            n160 = Unbundle By Name(w429) -> ("Image Ref"=w415:T9)
            n161 = Obtain Notifier(name (unnamed)="Display Module IMAQ Refs", notification data type=T9[] [], create if not found? (T)=FALSE) -> (notifier out=w422:refnum<notifier>, error out=w421:errorcluster)  [unwired: 1 in, 1 out]
            n162 = Get Notifier Status(notifier=w422, error in (no error)=w421) -> (notifier out=w423:refnum<notifier>, current notification=w425:T9[], error out=w424:errorcluster)  [unwired: 2 out]
            n163 = case shown="True" w413 {
              tunnel: w423 -> [w437 w447]
              tunnel: w424 -> [w431 w446]
              tunnel: w425 -> [w433 w449]
              tunnel: [w432 w448] -> w428
              tunnel: [w437 w447] -> w426
              tunnel: [w431 w446] -> w427
              tunnel: w415 -> [w430 w445]
              frame False {
                n164 = Equal?(x=w433, y=w430) -> (x = y?=w436:bool[])
                n165 = for {
                  tunnel: w436 -> [w444] mode=indexing
                  tunnel: [w443] -> w434
                  i -> [w443]
                  stop <- w444 stop-if-true
                }
                n166 = Or Array Elements(Boolean array=w436) -> (logical OR=w435:bool)
                n167 = case shown="False" w435 {
                  tunnel: w434 -> [_ w441]
                  tunnel: w433 -> [w438 w440]
                  tunnel: [w438 w439] -> w432
                  frame False {
                  }
                  frame True {
                    n168 = Delete From Array(array=w440, length=1, index=w441) -> (array with subset deleted=w439:T9[])  [unwired: 1 out]
                  }
                }
              }
              frame True {
                n169 = Build Array (concatenate)(w449, w445) -> (w448:T9[])
              }
            }
            n170 = Send Notification(notification=w428, notifier=w426, error in (no error)=w427) -> (notifier out=w420:refnum<notifier>, error out=w419:errorcluster)
            n171 = Release Notifier(notifier=w420, error in (no error)=w419) -> ()  [unwired: 1 in, 3 out]
          }
          event "Quit": Value Change {
            n172 = event-data() -> ("NewVal"=w455:bool)  [unwired: 1 in]
            n173 = Get Notifier Status(notifier=w453) -> (notifier out=w454:refnum<notifier>, current notification=w452:T7)  [unwired: 1 in, 3 out]
            n174 = Bundle By Name(cluster=w452, "Ximea Actions"=Ximea_Actions."Quit") -> (w451:T7)
            n175 = Send Notification(notification=w451, notifier=w454) -> ()  [unwired: 1 in, 2 out]
          }
        }
      }
      n176 = Release Notifier(notifier=w54, force destroy? (F)=TRUE) -> ()  [unwired: 1 in, 3 out]
    }
    frame Error {
      n177 = Release Notifier(notifier=w462, force destroy? (F)=TRUE, error in (no error)=w461) -> (error out=w460:errorcluster)  [unwired: 2 out]
      n178 = call "xiCam - CloseDevice.vi"("error in (no error)"=w460, "xiCam In"=w459) -> ("error out"=w458:errorcluster)  [unwired: 9 in]
      n179 = call "IMAQ Dispose"("Image"=w456, "error in (no error)"=w458) -> ("error out"=w457:errorcluster)  [unwired: 4 in]
      n180 = Unbundle By Name(w457) -> ("source"=w464:string)
      n181 = call <vilib>:"Space Constant.vi"() -> ("String"=w467:string)
      n182 = Concatenate Strings(w463, w467, "Device Error." ("string"), "\r", w464) -> (w468:string)
      n183 = One Button Dialog(message=w468) -> ()  [unwired: 1 in, 1 out]
    }
  }
